vi "Miscalleneous.vi"() -> ()   [LabVIEW 2014]
panel:
  out "Translation Motion?":bool
  in  "Magnetometer Start angle":dbl
  in  "Start Robot Angle":dbl
  out "Step Deployment Completed Last Cycle":bool
  out "Scissors Deployment finished":bool
  out "Setpoint Reached":bool
  out "Can Completed Loading Last Cycle":bool
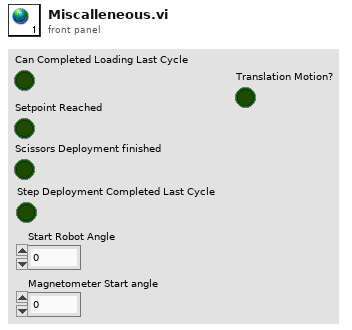
[diagram p1: front panel]
diagram:
